vi "File Parser.vi"(8 "error in (no error)":errorcluster) -> (0 "error out":errorcluster, 2 "Morse-Letter Map (output 2)":map{string, string}(c390), 3 "Letter-Morse Map (output 1)":map{string, string}(c390))   [LabVIEW 2022 SP3]
uses:
  <vilib>/Utility/file.llb/Read Delimited Spreadsheet (string).vi
panel:
  out "Morse Array":string[](array[string])
  out "Letter Array":string[](array[string])
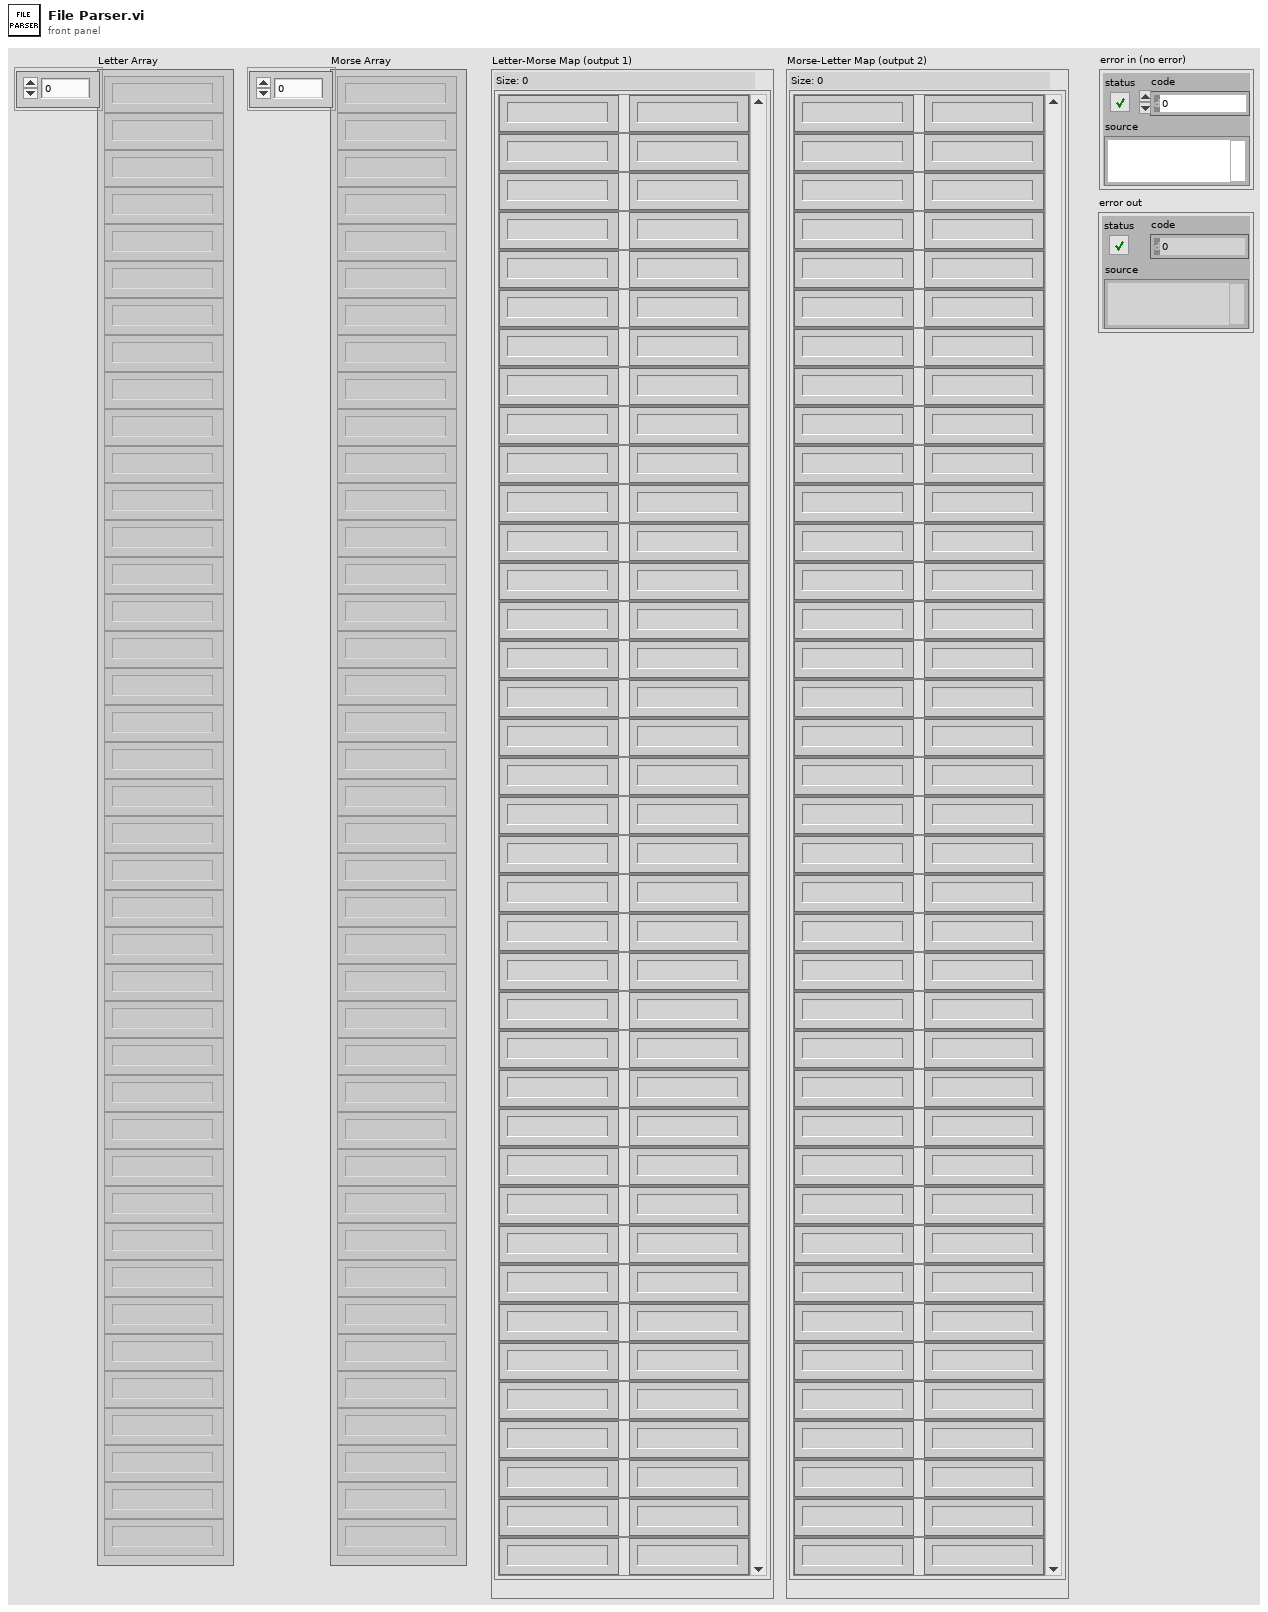
[diagram p1: front panel]
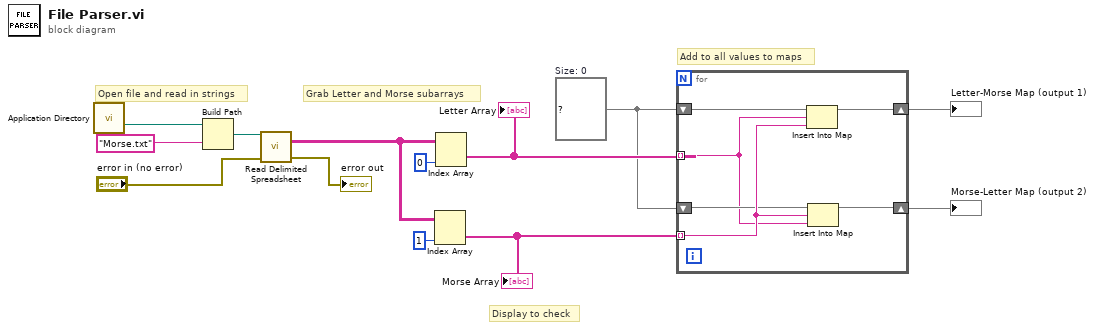
[diagram p0: block diagram]
diagram:
  w1 = map{string, string} {}  # Size: 0
  # "Add to all values to maps"
  # "Display to check"
  # "Grab Letter and Morse subarrays"
  # "Open file and read in strings"
  n1 = call <vilib>:"Application Directory.vi"() -> ("Application Directory"=w4:path)
  n2 = Build Path(base path=w4, name or relative path="Morse.txt") -> (appended path=w2:path)
  n3 = call-poly <vilib>:"Read Delimited Spreadsheet.vi"("file path (dialog if empty)"=w2, "error in (no error)"="error in (no error)") -> ("all rows"=w12:string[][], "error out"=→"error out":errorcluster)  [unwired: 8 in, 4 out]
  n4 = Index Array(array=w12, index (col)=1 ("disabled index (col)")) -> (element=w10:string[])  [unwired: 1 in]
  "Morse Array" <- w10
  n5 = Index Array(array=w12, index (col)=0 ("disabled index (col)")) -> (element=w9:string[])  [unwired: 1 in]
  "Letter Array" <- w9
  n6 = for {
    tunnel: w10 -> [w17] mode=indexing
    tunnel: w9 -> [w14] mode=indexing
    shift-right: [w19] -> w8
    shift-left: w1 -> [w18]
    shift-right: [w15] -> w7
    shift-left: w1 -> [w16]
    n7 = Insert Into Map(map in=w18, key=w14, value=w17) -> (map out=w19:map{string, string})  [unwired: 2 out]
    n8 = Insert Into Map(map in=w16, key=w17, value=w14) -> (map out=w15:map{string, string})  [unwired: 2 out]
  }
  "Letter-Morse Map (output 1)" <- w8
  "Morse-Letter Map (output 2)" <- w7
